vi "Add ByteArray.vi"(8 "error in":errorcluster, 10 "bytes":u8[](array[numeric]) format="%02x", 11 "Buffer":refnum<data-value>) -> (0 "error out":errorcluster, 3 "Buffer":refnum<data-value>)   [LabVIEW 2013, in "ByteBuffer.lvclass"]
doc: "This VI allows to input an array into the buffer. The location in the buffer is updated automatically.\n\nIf the input array is larger than the buffer then just take last elements of the input array and save them in the buffer. Also give a warning that this happened."
uses:
  ByteBuffer.lvclass
  VariantBuffer/VariantBuffer.lvclass
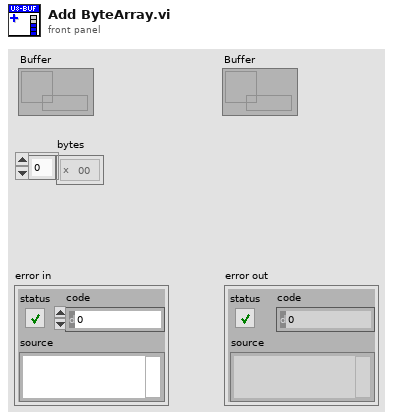
[diagram p1: front panel]
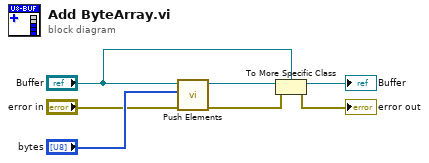
[diagram p0: block diagram]
diagram:
  n1 = call "Push Elements.vi"("error in"="error in", "elements"="bytes", "Buffer in"="Buffer") -> ("error out"=w2:errorcluster, "Buffer"=w5:refnum<data-value>)  [unwired: 7 in]
  n2 = To More Specific Class(target class="Buffer", reference=w5, error in=w2) -> (specific class reference=→"Buffer":refnum<data-value>, error out=→"error out":errorcluster)
